vi "DatabaseUISpecificInfo.vi"(0 "RequestActor":refnum<class "RequestRestUI.lvclass">, 11 "error in (no error)":errorcluster) -> (4 "RequestActor out":refnum<class "RequestRestUI.lvclass">, 6 "TableName":string, 8 "TableItems":string[](array[string]), 10 "TableItemInfo":T2[](array[typedef]), 15 "error out":errorcluster)   [LabVIEW 2015, in "UserManagement.lvlib" / "RequestRestMember.lvclass"]
uses:
  UserManagement/Emengency/RequestRestMember.lvclass
  <vilib>/addons/database/Auxilliary.llb/DB Tools DataTypes.ctl
  <vilib>/addons/database/NI_Database_API.lvlib
  <vilib>/addons/database/Auxilliary.llb/DB Tools Column Info.ctl
  typedef/RequestRestInfo.ctl
  RequestRestUI.lvclass
panel:
  in  "请假内容":T1
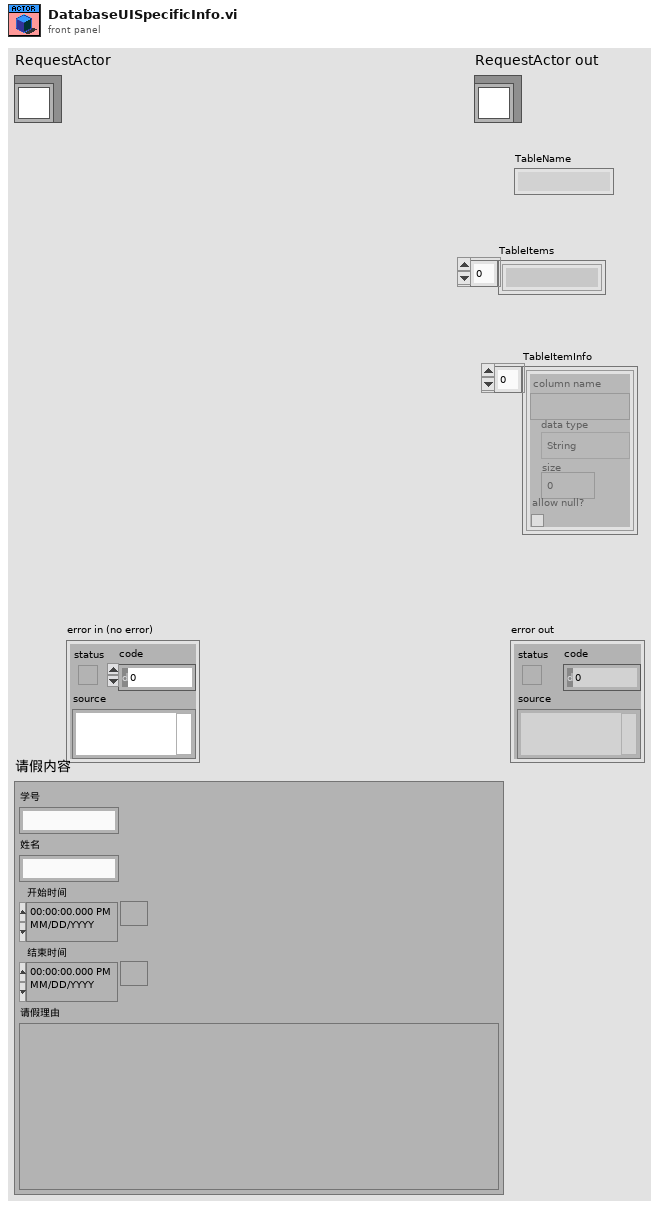
[diagram p1: front panel]
types:
  T1 = typedef "RequestRestUI.lvclass/RequestRestInfo.ctl" = cluster{"学号":string, "姓名":string, "开始时间":timestamp, "结束时间":timestamp, "请假理由":string}
  T2 = typedef "NI_Database_API.lvlib/DB Tools Column Info.ctl" = cluster{"column name":string, "data type":T3, "size":i32, "allow null?":bool}
  T3 = typedef "NI_Database_API.lvlib/DB Tools DataTypes.ctl" = enum16{"String", "Long (I32)", "Single (SGL)", "Double (DBL)", "Date/Time", "Binary"}
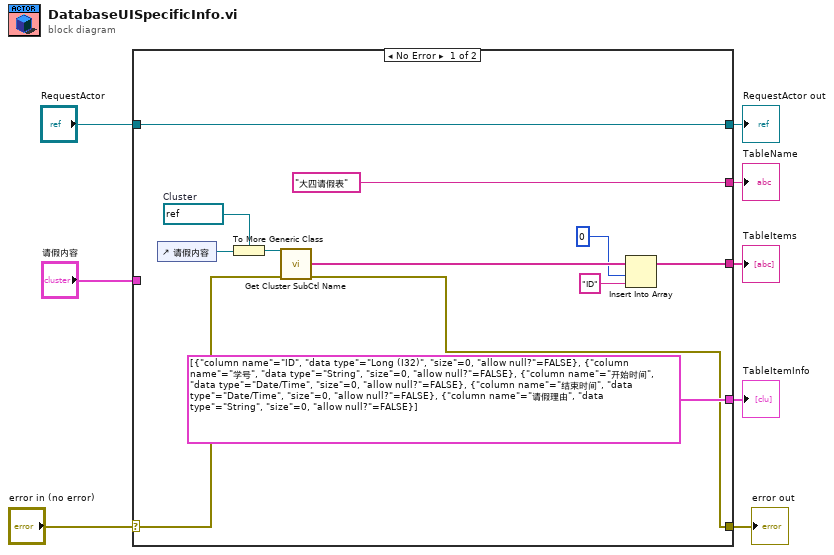
[diagram p0: block diagram]
diagram:
  n1 = case shown="No Error" "error in (no error)" {
    selector: "error in (no error)" -> [w15 w22]
    tunnel: [w10 w22] -> w7
    tunnel: ["大四请假表" _] -> w6
    tunnel: [T2[] [{"column name"="ID", "data type"=enum."Long (I32)", "size"=0, "allow null?"=FALSE}, {"column name"="学号", "data type"=enum."String", "size"=0, "allow null?"=FALSE}, {"column name"="开始时间", "data type"=enum."Date/Time", "size"=0, "allow null?"=FALSE}, {"column name"="结束时间", "data type"=enum."Date/Time", "size"=0, "allow null?"=FALSE}, {"column name"="请假理由", "data type"=enum."String", "size"=0, "allow null?"=FALSE}] ("column information") _] -> w5
    tunnel: "请假内容" -> [_ _]
    tunnel: [w11 _] -> w3
    tunnel: "RequestActor" -> [w9 w21]
    tunnel: [w9 w21] -> w1
    frame No Error {
      w16 = refnum<vi> refnum  # Cluster
      n2 = control-ref of="请假内容"() -> (w18:refnum<vi>)
      n3 = To More Generic Class(target class=w16, reference=w18) -> (generic class reference=w17:refnum<vi>)
      n4 = call "Get Cluster SubCtl Name.vi"("error in (no error)"=w15, "Clust Ref"=w17) -> ("error out"=w10:errorcluster, "CtlName"=w14:string[])  [unwired: 7 in, 1 out]
      n5 = Insert Into Array(array=w14, index=0, new element="ID" ("new element/subarray")) -> (w11:string[])
    }
    frame Error {
    }
  }
  "error out" <- w7
  "TableName" <- w6
  "TableItems" <- w3
  "TableItemInfo" <- w5
  "RequestActor out" <- w1
